vi "fgvEvent.vi"(8 "error in (no error)":errorcluster, 9 "Cmd":string, 10 "EventRefNum":refnum<event-registration>, 11 "eventData":refnum<user-event>) -> (0 "error out":errorcluster, 2 "EventRefNum Out":refnum<event-registration>, 3 "eventData Out":refnum<user-event>)   [LabVIEW 2013, in "CONTROLLER.lvclass"]
uses:
  CONTROLLER.lvclass
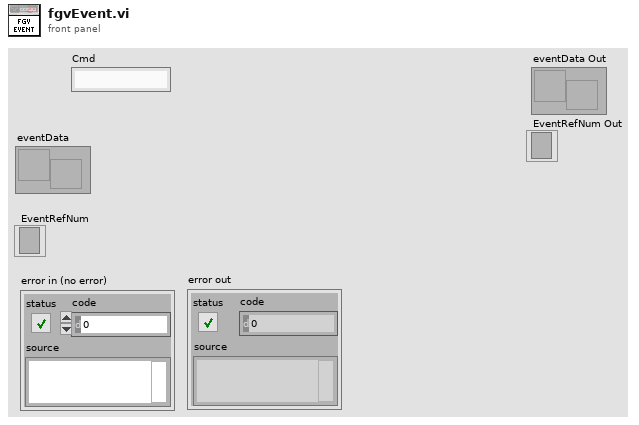
[diagram p1: front panel]
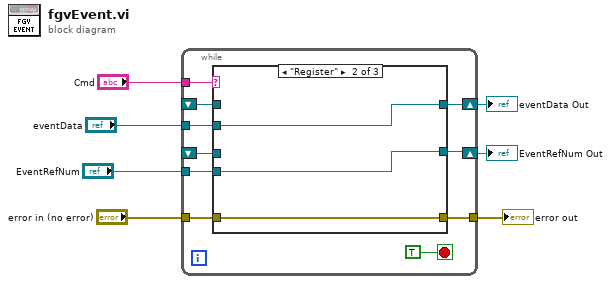
[diagram p0: block diagram]
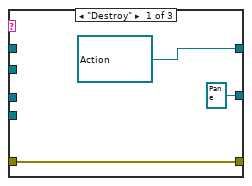
[diagram p2: hidden frame]
diagram:
  n1 = while {
    tunnel: "Cmd" -> [w16]
    shift-right: [w15] -> w4
    shift-left: _ -> [w10]
    tunnel: "eventData" -> [w14]
    shift-right: [w11] -> w3
    shift-left: _ -> [w13]
    tunnel: "EventRefNum" -> [w12]
    tunnel: "error in (no error)" -> [w9]
    tunnel: [w8] -> w1
    stop <- TRUE stop-if-true
    n2 = case shown="\"Register\"" w16 {
      tunnel: [refnum<user-event> refnum ("eventData") w23 w26] -> w15
      tunnel: w14 -> [_ w23 _]
      tunnel: w13 -> [_ _ w25]
      tunnel: [refnum<event-registration> refnum ("EventRefNum") w22 w25] -> w11
      tunnel: w12 -> [_ w22 _]
      tunnel: w10 -> [_ _ w26]
      tunnel: w9 -> [w18 w21 w24]
      tunnel: [w18 w21 w24] -> w8
      frame "Destroy" {
      }
      frame "Register" {
      }
      frame "Read", Default {
      }
    }
  }
  "eventData Out" <- w4
  "EventRefNum Out" <- w3
  "error out" <- w1
